vi "Find_ball.vi"(0 "Image Input":T1, 3 "error in (no error)":errorcluster) -> (4 "Image Out":T1(plugin-control), 5 "Plate coordinates":sgl[](array[numeric]), 6 "Ball Coordinates":cluster{"x":sgl, "y":sgl}, 7 "error out":errorcluster)   [LabVIEW 2021]
uses:
  <vilib>/vision/Image Controls.llb/IMAQ Image.ctl
  <vilib>/vision/NI_Vision_Development_Module.lvlib
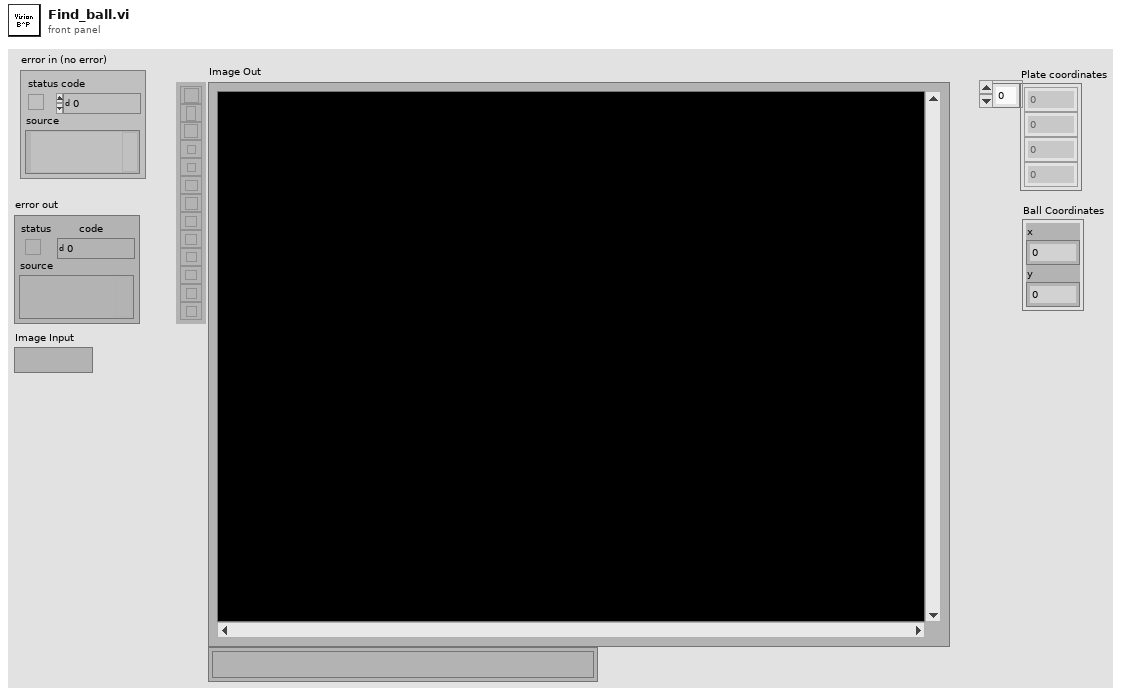
[diagram p1: front panel]
types:
  T1 = typedef "IMAQ Image.ctl" = refnum<image>
  T2 = cluster{"Feature":u32, "Points IDs":cluster{"GUID":string, "Index":i32}[]}[]
  T3 = typedef "Image Type" = u32
  T4 = cluster{"Global Rectangle":i32[], "Contours":cluster{"ID":enum32{"External", "Internal"}, "Type":u32, "Coordinates":i32[]}[]}
  T5 = cluster{"Show Search Area":bool, "Show Search Lines":bool, "Show Edges Found":bool, "Show Result":bool}
  T6 = cluster{"Number of Lines":i32, "Type":enum32{"First Edge Rake", "Best Edge Rake", "Hough Edge Rake", "First Edge Projection", "Best Edge Projection"}, "Min. Score":dbl, "Max. Score":dbl, "Orientation":dbl, "Angle Range":dbl, "Angle Tolerance":dbl, "Step Size":u32, "Min. SNR (db)":dbl, "Min. Points (%)":dbl, "Hough Iterations":i32}
  T7 = cluster{"Edge Polarity":u32, "Kernel Size":u32, "Width":u32, "Minimum Edge Strength":sgl, "Interpolation Type":enum32{"Zero Order", "Bilinear", "Quadratic", "Cubic", "Bilinear Fixed"}, "Data Processing Method":enum32{"Average", "Median"}}
  T8 = cluster{"Origin Pixel":cluster{"X":sgl, "Y":sgl}, "X Axis Pixel":cluster{"X":sgl, "Y":sgl}, "Axis Reference":u32}
  T9 = cluster{"Point1 (Pixels)":cluster{"X":sgl, "Y":sgl}, "Point2 (Pixels)":cluster{"X":sgl, "Y":sgl}, "Point1 (Real-World)":cluster{"X":sgl, "Y":sgl}, "Point2 (Real-World)":cluster{"X":sgl, "Y":sgl}, "Angle (Pixel)":dbl, "Angle (Real-World)":dbl, "Score":dbl, "Straightness":dbl, "Average SNR (db)":dbl, "Calibration Valid":bool}[]
  T10 = typedef "Search Line.ctl" = cluster{"Start Point":cluster{"X":sgl, "Y":sgl}, "End Point":cluster{"X":sgl, "Y":sgl}, "Edge Info":T11[], "Edge Map":dbl[], "Calibration Valid":bool}
  T11 = typedef "Edge New.ctl" = cluster{"Location (Pixel)":cluster{"X":sgl, "Y":sgl}, "Location (Real-World)":cluster{"X":sgl, "Y":sgl}, "Distance (Pixel)":dbl, "Distance (Real-World)":dbl, "Strength":dbl, "Noise":dbl, "Rising?":bool}
  T12 = cluster{"Straight Edges":cluster{"Point1 (Pixels)":cluster{"X":sgl, "Y":sgl}, "Point2 (Pixels)":cluster{"X":sgl, "Y":sgl}, "Point1 (Real-World)":cluster{"X":sgl, "Y":sgl}, "Point2 (Real-World)":cluster{"X":sgl, "Y":sgl}, "Angle (Pixel)":dbl, "Angle (Real-World)":dbl, "Score":dbl, "Straightness":dbl, "Average SNR (db)":dbl, "Calibration Valid":bool}[], "Search Lines Information":T10[], "Used Edges":cluster{"Edge Information":T11[]}[]}
  T13 = cluster{"Position":cluster{"x":sgl, "y":sgl}, "Angle":sgl, "Scale":sgl, "Score":sgl, "Bounding Box":cluster{"x":sgl, "y":sgl}[]}[]
  T14 = cluster{"Position":cluster{"x":sgl, "y":sgl}, "Angle":sgl, "Scale":sgl, "Score":sgl, "Bounding Box":cluster{"x":sgl, "y":sgl}[]}
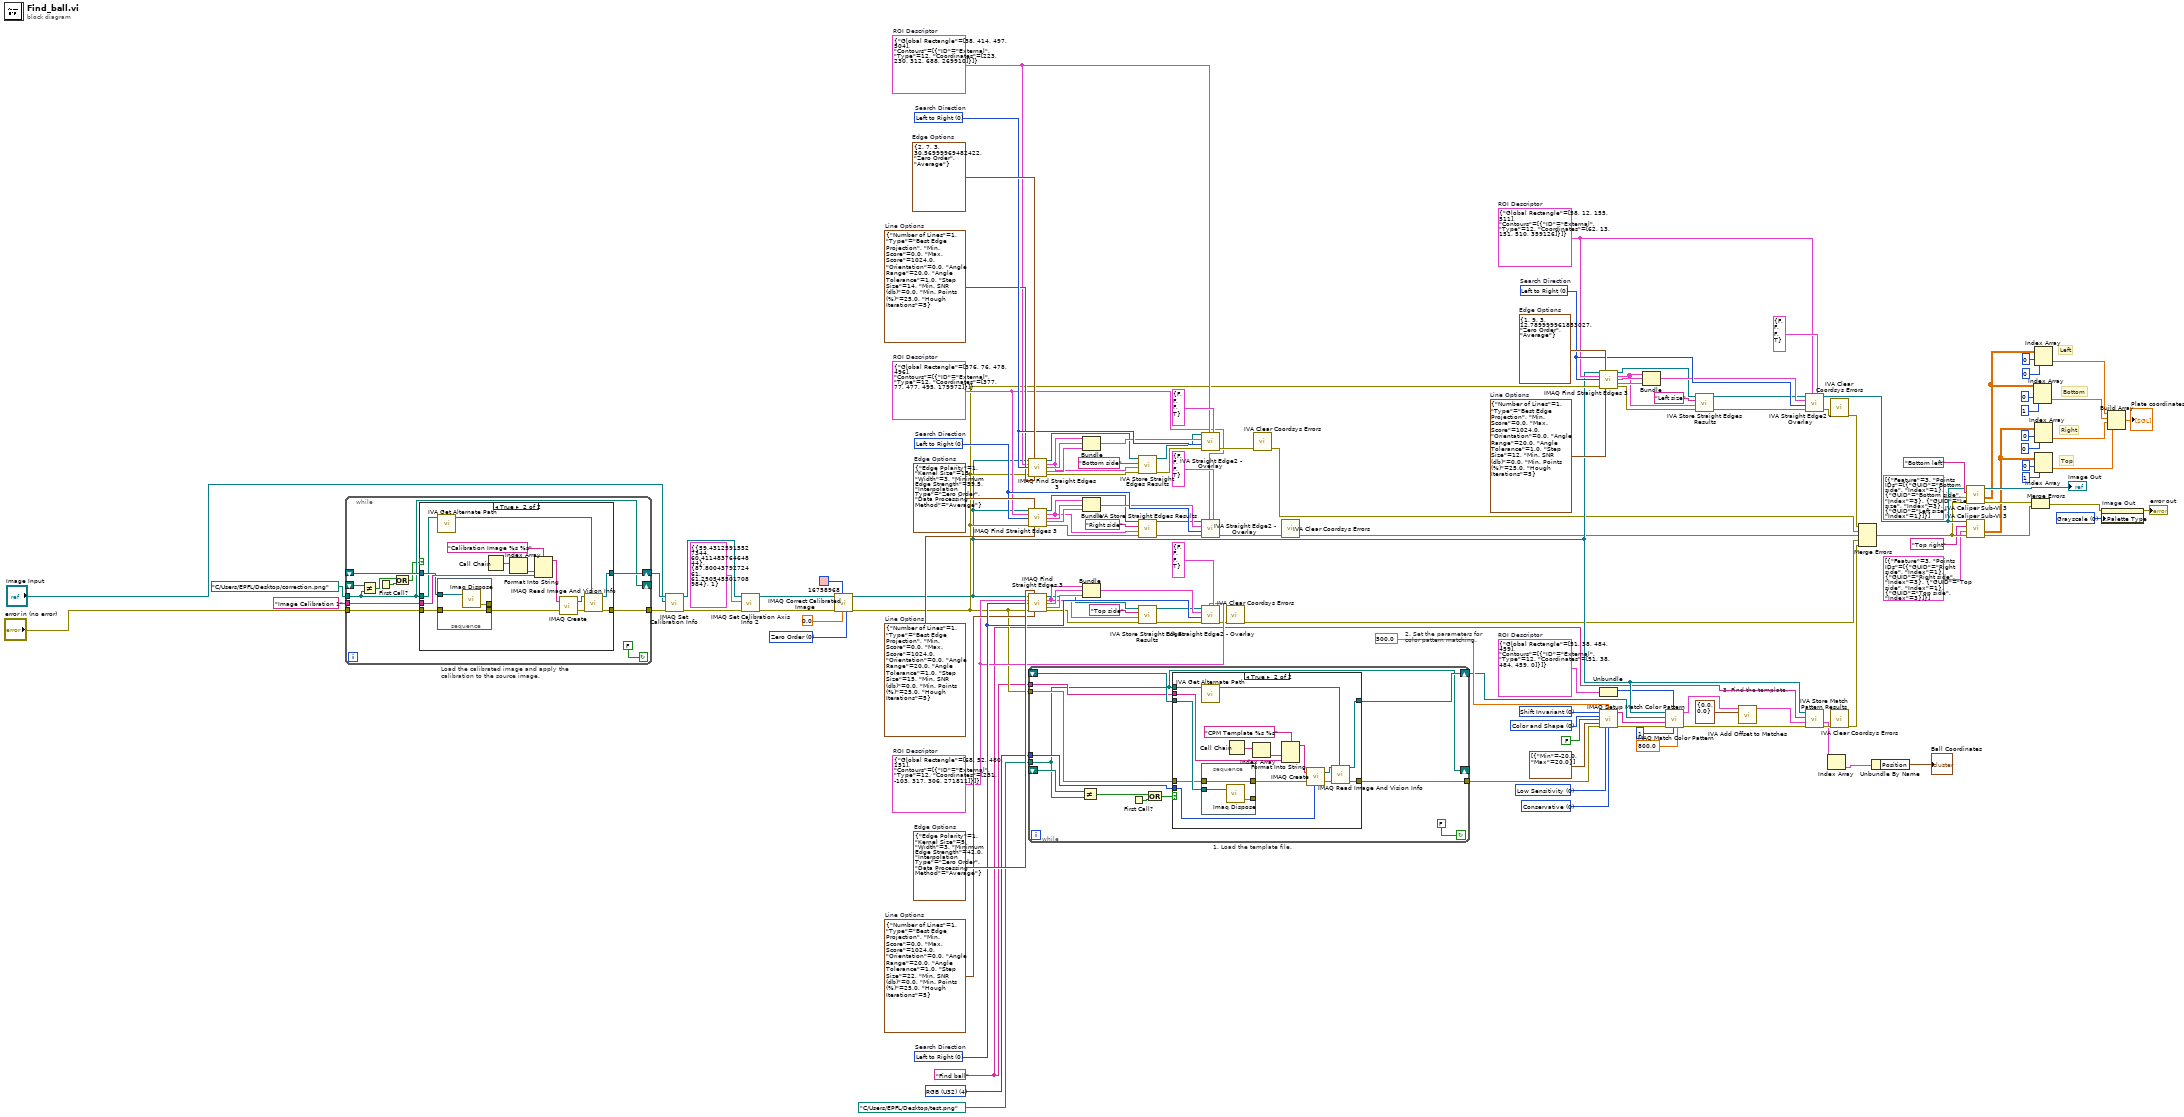
[diagram p0: block diagram]
diagram:
  w21 = u32 0 items=["Grayscale", "Binary", "Gradient", "Rainbow", "Temperature", "User Defined", "Binary 16 Bit", "Gradient 16 Bit", "Rainbow 16 Bit", "Temperature 16 Bit", "User Defined 16 Bit"] ("Palette Type")
  w45 = "Find ball" ("Step Name")
  w53 = T3 4 items=["Grayscale (U8)", "Grayscale (I16)", "Grayscale (SGL)", "Complex (CSG)", "RGB (U32)", "HSL (U32)", "RGB (U64)"] ("Image Type")
  w56 = u32 0 items=["Conservative", "Balance", "Aggressive", "Very Aggressive"] ("Search Strategy")
  w57 = u32 0 items=["Low Sensitivity", "Medium Sensitivity", "High Sensitivity"] ("Color Sensitivity")
  w59 = u32 0 items=["Color and Shape", "Color", "Shape"] ("Match Feature Mode")
  w60 = u32 0 items=["Shift Invariant", "Rotation Invariant"] ("Match Mode")
  w50 = T4 {"Global Rectangle"=[51, 38, 484, 459], "Contours"=[{"ID"=enum."External", "Type"=12, "Coordinates"=[51, 38, 484, 459, 0]}]}  # ROI Descriptor
  w75 = T6 {"Number of Lines"=1, "Type"=enum."Best Edge Projection", "Min. Score"=0.0, "Max. Score"=1024.0, "Orientation"=0.0, "Angle Range"=20.0, "Angle Tolerance"=1.0, "Step Size"=22, "Min. SNR (db)"=0.0, "Min. Points (%)"=25.0, "Hough Iterations"=5}  # Line Options
  w76 = u32 0 items=["Left to Right", "Right to Left", "Top to Bottom", "Bottom to Top"]  # Search Direction
  w77 = T7 {"Edge Polarity"=1, "Kernel Size"=5, "Width"=3, "Minimum Edge Strength"=42.0, "Interpolation Type"=enum."Zero Order", "Data Processing Method"=enum."Average"}  # Edge Options
  w70 = T4 {"Global Rectangle"=[68, 52, 480, 151], "Contours"=[{"ID"=enum."External", "Type"=12, "Coordinates"=[231, -103, 317, 306, 271811]}]}  # ROI Descriptor
  w90 = T6 {"Number of Lines"=1, "Type"=enum."Best Edge Projection", "Min. Score"=0.0, "Max. Score"=1024.0, "Orientation"=0.0, "Angle Range"=20.0, "Angle Tolerance"=1.0, "Step Size"=15, "Min. SNR (db)"=0.0, "Min. Points (%)"=25.0, "Hough Iterations"=5}  # Line Options
  w91 = u32 0 items=["Left to Right", "Right to Left", "Top to Bottom", "Bottom to Top"]  # Search Direction
  w92 = T7 {"Edge Polarity"=1, "Kernel Size"=15, "Width"=3, "Minimum Edge Strength"=59.5, "Interpolation Type"=enum."Zero Order", "Data Processing Method"=enum."Average"}  # Edge Options
  w85 = T4 {"Global Rectangle"=[376, 76, 478, 496], "Contours"=[{"ID"=enum."External", "Type"=12, "Coordinates"=[377, 77, 477, 495, 179972]}]}  # ROI Descriptor
  w105 = T6 {"Number of Lines"=1, "Type"=enum."Best Edge Projection", "Min. Score"=0.0, "Max. Score"=1024.0, "Orientation"=0.0, "Angle Range"=20.0, "Angle Tolerance"=1.0, "Step Size"=14, "Min. SNR (db)"=0.0, "Min. Points (%)"=25.0, "Hough Iterations"=5}  # Line Options
  w106 = u32 0 items=["Left to Right", "Right to Left", "Top to Bottom", "Bottom to Top"]  # Search Direction
  w107 = T7 {"Edge Polarity"=2, "Kernel Size"=7, "Width"=3, "Minimum Edge Strength"=30.57, "Interpolation Type"=enum."Zero Order", "Data Processing Method"=enum."Average"}  # Edge Options
  w100 = T4 {"Global Rectangle"=[38, 414, 497, 504], "Contours"=[{"ID"=enum."External", "Type"=12, "Coordinates"=[223, 230, 312, 688, 269910]}]}  # ROI Descriptor
  w120 = T6 {"Number of Lines"=1, "Type"=enum."Best Edge Projection", "Min. Score"=0.0, "Max. Score"=1024.0, "Orientation"=0.0, "Angle Range"=20.0, "Angle Tolerance"=1.0, "Step Size"=12, "Min. SNR (db)"=0.0, "Min. Points (%)"=25.0, "Hough Iterations"=5}  # Line Options
  w121 = u32 0 items=["Left to Right", "Right to Left", "Top to Bottom", "Bottom to Top"]  # Search Direction
  w122 = T7 {"Edge Polarity"=1, "Kernel Size"=9, "Width"=3, "Minimum Edge Strength"=12.79, "Interpolation Type"=enum."Zero Order", "Data Processing Method"=enum."Average"}  # Edge Options
  w115 = T4 {"Global Rectangle"=[58, 12, 155, 511], "Contours"=[{"ID"=enum."External", "Type"=12, "Coordinates"=[62, 13, 151, 510, 359126]}]}  # ROI Descriptor
  w127 = u32 0 items=["Zero Order", "Bi-Linear", "Quadratic", "Cubic Spline"] ("Interpolation Type")
  # "Top"
  # "Right"
  # "Bottom"
  # "Left"
  # "2. Set the parameters for\ncolor pattern matching."
  # "3. Find the template."
  n1 = while "Load the calibrated image and apply the calibration to the source image." {
    shift-right: [w145] -> w133
    shift-left: _ -> [w144]
    tunnel: [w142] -> w132
    tunnel: "error in (no error)" -> [w141]
    tunnel: path "C:/Users/EPFL/Desktop/correction.png" ("File Path") -> [w138]
    tunnel: "Image Calibration 1" ("Step Name") -> [w140]
    shift-right: [w138] -> _
    shift-left: _ -> [w139]
    stop <- FALSE continue-if-true
    n2 = Not Equal?(x=w139, y=w138) -> (x != y?=w136:bool)
    n3 = First Call?() -> (First Call?: T/F=w137:bool)
    n4 = Or(x=w136, y=w137) -> (x .or. y?=w135:bool)
    n5 = case shown="True" w135 {
      tunnel: [w147 w159] -> w145
      tunnel: w144 -> [w147 w151]
      tunnel: [w146 w156] -> w142
      tunnel: w141 -> [w146 w152]
      tunnel: w138 -> [_ w149]
      tunnel: w140 -> [_ w153]
      frame False {
      }
      frame True {
        n6 = call <vilib>:"IVA Get Alternate Path.vi"("Path In"=w149) -> ("Path Out"=w148:path)  [unwired: 10 out]
        n7 = stacked-sequence {
          tunnel: w152 -> [w163]
          tunnel: w151 -> [w164]
          tunnel: [w163] -> w150
          tunnel: [w162] -> _
          frame #0 {
            n8 = call "Imaq Dispose"("Image"=w164) -> ("error out"=w162:errorcluster)  [unwired: 2 in, 3 out]
          }
        }
        n9 = Call Chain() -> (call chain=w155:string[])
        n10 = Index Array(array=w155) -> (element=w154:string)  [unwired: 1 in]
        n11 = Format Into String(format string="Calibration Image %s %s" ("Image Name"), w154, w153) -> (resulting string=w161:string)  [unwired: 2 in, 1 out]
        n12 = call "IMAQ Create"("Image Name"=w161, "error in (no error)"=w150) -> ("New Image"=w158:T1, "error out"=w157:errorcluster)  [unwired: 2 in, 1 out]
        n13 = call "IMAQ Read Image And Vision Info"("File Path"=w148, "error in (no error)"=w157, "Image"=w158) -> ("error out"=w156:errorcluster, "Image Out"=w159:T1)  [unwired: 1 in, 6 out]
      }
    }
  }
  n14 = call "IMAQ Set Calibration Info"("error in (no error)"=w132, "Image Dst"="Image Input", "Image Src"=w133) -> ("error out"=w129:errorcluster, "Calibrated Image"=w130:T1)  [unwired: 1 in, 6 out]
  n15 = call-poly "IMAQ Set Calibration Axis Info 2"("error in (no error)"=w129, "Calibration Axis Info"=T8 {"Origin Pixel"={"X"=59.43126, "Y"=60.411484}, "X Axis Pixel"={"X"=87.80044, "Y"=61.250546}, "Axis Reference"=1}, "Calibration Template Image In"=w130) -> ("error out"=w125:errorcluster, "Calibration Template Image Out"=w126:T1)  [unwired: 7 out]
  n16 = call "IMAQ Correct Calibrated Image"("Interpolation Type"=w127, "Replace Value"=sgl 0.0, "Color Replace Value"=u32 16758968, "error in (no error)"=w125, "Image Src"=w126) -> ("error out"=w49:errorcluster, "Corrected Image"=w46:T1)  [unwired: 2 in, 3 out]
  n17 = call "IMAQ Find Straight Edges 3"("Image"=w46, "Edge Options"=w107, "ROI Descriptor"=w100, "Search Direction"=w106, "error in (no error)"=w49, "Line Options"=w105) -> ("Image (duplicate)"=w97:T1, "Straight Edges"=w98:T9, "Search Lines Information"=w102:T10[], "Used Edges"=w103:cluster{"Edge Information":T11[]}[], "error out"=w95:errorcluster)  [unwired: 1 in, 4 out]
  n18 = call "IMAQ Find Straight Edges 3"("Image"=w46, "Edge Options"=w92, "ROI Descriptor"=w85, "Search Direction"=w91, "error in (no error)"=w49, "Line Options"=w90) -> ("Image (duplicate)"=w82:T1, "Straight Edges"=w83:T9, "Search Lines Information"=w87:T10[], "Used Edges"=w88:cluster{"Edge Information":T11[]}[], "error out"=w80:errorcluster)  [unwired: 1 in, 4 out]
  n19 = call "IMAQ Find Straight Edges 3"("Image"=w46, "Edge Options"=w77, "ROI Descriptor"=w70, "Search Direction"=w76, "error in (no error)"=w49, "Line Options"=w75) -> ("Image (duplicate)"=w67:T1, "Straight Edges"=w68:T9, "Search Lines Information"=w72:T10[], "Used Edges"=w73:cluster{"Edge Information":T11[]}[], "error out"=w65:errorcluster)  [unwired: 1 in, 4 out]
  n20 = while "1. Load the template file." {
    shift-right: [w176] -> w40
    shift-left: _ -> [w175]
    tunnel: [w173] -> w39
    tunnel: w49 -> [w172]
    tunnel: path "C:/Users/EPFL/Desktop/test.png" ("File Path") -> [w168]
    tunnel: w53 -> [w171]
    tunnel: w45 -> [w170]
    shift-right: [w168] -> _
    shift-left: _ -> [w169]
    stop <- FALSE continue-if-true
    n21 = Not Equal?(x=w169, y=w168) -> (x != y?=w166:bool)
    n22 = First Call?() -> (First Call?: T/F=w167:bool)
    n23 = Or(x=w166, y=w167) -> (x .or. y?=w165:bool)
    n24 = case shown="True" w165 {
      tunnel: [w178 w191] -> w176
      tunnel: w175 -> [w178 w183]
      tunnel: [w177 w188] -> w173
      tunnel: w172 -> [w177 w182]
      tunnel: w168 -> [_ w180]
      tunnel: w171 -> [_ w187]
      tunnel: w170 -> [_ w184]
      frame False {
      }
      frame True {
        n25 = call <vilib>:"IVA Get Alternate Path.vi"("Path In"=w180) -> ("Path Out"=w179:path)  [unwired: 10 out]
        n26 = stacked-sequence {
          tunnel: w183 -> [w196]
          tunnel: w182 -> [w195]
          tunnel: [w195] -> w181
          tunnel: [w194] -> _
          frame #0 {
            n27 = call "Imaq Dispose"("Image"=w196) -> ("error out"=w194:errorcluster)  [unwired: 2 in, 3 out]
          }
        }
        n28 = Call Chain() -> (call chain=w186:string[])
        n29 = Index Array(array=w186) -> (element=w185:string)  [unwired: 1 in]
        n30 = Format Into String(format string="CPM Template %s %s" ("Image Name"), w185, w184) -> (resulting string=w193:string)  [unwired: 2 in, 1 out]
        n31 = call "IMAQ Create"("Image Name"=w193, "Image Type"=w187, "error in (no error)"=w181) -> ("New Image"=w190:T1, "error out"=w189:errorcluster)  [unwired: 1 in, 1 out]
        n32 = call "IMAQ Read Image And Vision Info"("File Path"=w179, "error in (no error)"=w189, "Image"=w190) -> ("error out"=w188:errorcluster, "Image Out"=w191:T1)  [unwired: 1 in, 6 out]
      }
    }
  }
  n33 = Bundle("Straight Edges"=w98, "Search Lines Information"=w102, "Used Edges"=w103) -> (w99:T12)  [unwired: 1 out]
  n34 = Bundle("Straight Edges"=w83, "Search Lines Information"=w87, "Used Edges"=w88) -> (w84:T12)  [unwired: 1 out]
  n35 = Bundle("Straight Edges"=w68, "Search Lines Information"=w72, "Used Edges"=w73) -> (w69:T12)  [unwired: 1 out]
  n36 = call <vilib>:"IVA Store Straight Edges Results.vi"("error in (no error)"=w95, "Straight Edges"=w98, "Step Name"="Bottom side", "Image in"=w97) -> ("error out"=w94:errorcluster, "Image dup"=w96:T1)  [unwired: 6 out]
  n37 = call <vilib>:"IVA Store Straight Edges Results.vi"("error in (no error)"=w80, "Straight Edges"=w83, "Step Name"="Right side", "Image in"=w82) -> ("error out"=w79:errorcluster, "Image dup"=w81:T1)  [unwired: 6 out]
  n38 = call <vilib>:"IVA Store Straight Edges Results.vi"("error in (no error)"=w65, "Straight Edges"=w68, "Step Name"="Top side", "Image in"=w67) -> ("error out"=w64:errorcluster, "Image dup"=w66:T1)  [unwired: 6 out]
  n39 = call <vilib>:"IVA Straight Edge2 - Overlay.vi"("Setup"=T5 {"Show Search Area"=FALSE, "Show Search Lines"=FALSE, "Show Edges Found"=FALSE, "Show Result"=TRUE}, "Search Area"=w100, "error in (no error)"=w94, "Scan Direction"=w106, "Edge Results"=w99, "Image In"=w96) -> ("error out"=w93:errorcluster)  [unwired: 1 in, 4 out]
  n40 = call <vilib>:"IVA Straight Edge2 - Overlay.vi"("Setup"=T5 {"Show Search Area"=FALSE, "Show Search Lines"=FALSE, "Show Edges Found"=FALSE, "Show Result"=TRUE}, "Search Area"=w85, "error in (no error)"=w79, "Scan Direction"=w91, "Edge Results"=w84, "Image In"=w81) -> ("error out"=w78:errorcluster)  [unwired: 1 in, 4 out]
  n41 = call <vilib>:"IVA Straight Edge2 - Overlay.vi"("Setup"=T5 {"Show Search Area"=FALSE, "Show Search Lines"=FALSE, "Show Edges Found"=FALSE, "Show Result"=TRUE}, "Search Area"=w70, "error in (no error)"=w64, "Scan Direction"=w76, "Edge Results"=w69, "Image In"=w66) -> ("error out"=w63:errorcluster)  [unwired: 1 in, 4 out]
  n42 = call <vilib>:"IVA Clear Coordsys Errors.vi"("error in (no error)"=w63) -> ("error out"=w34:errorcluster)  [unwired: 10 in]
  n43 = call <vilib>:"IVA Clear Coordsys Errors.vi"("error in (no error)"=w93) -> ("error out"=w36:errorcluster)  [unwired: 10 in]
  n44 = call <vilib>:"IVA Clear Coordsys Errors.vi"("error in (no error)"=w78) -> ("error out"=w35:errorcluster)  [unwired: 10 in]
  n45 = call "IMAQ Find Straight Edges 3"("Image"=w46, "Edge Options"=w122, "ROI Descriptor"=w115, "Search Direction"=w121, "error in (no error)"=w49, "Line Options"=w120) -> ("Image (duplicate)"=w112:T1, "Straight Edges"=w113:T9, "Search Lines Information"=w117:T10[], "Used Edges"=w118:cluster{"Edge Information":T11[]}[], "error out"=w110:errorcluster)  [unwired: 1 in, 4 out]
  n46 = Unbundle(w50) -> ("Global Rectangle"=w41:i32[])  [unwired: 1 out]
  n47 = call "IMAQ Setup Match Color Pattern"("Match Mode"=w60, "Color Score Weight"=sgl 500.0, "Match Feature Mode"=w59, "Subpixel Accuracy"=FALSE, "Rotation Angle Ranges (degrees)"=cluster{"Min":sgl, "Max":sgl}[] [{"Min"=-20.0, "Max"=20.0}], "error in (no error)"=w39, "Color Sensitivity"=w57, "Search Strategy"=w56) -> ("Match Color Pattern Setup Data"=w44:string, "error out"=w43:errorcluster)  [unwired: 1 in, 5 out]
  n48 = Bundle("Straight Edges"=w113, "Search Lines Information"=w117, "Used Edges"=w118) -> (w114:T12)  [unwired: 1 out]
  n49 = call "IMAQ Match Color Pattern"("Minimum Match Score"=sgl 800.0, "Number of Matches Requested"=1, "Optional Rectangle"=w41, "error in (no error)"=w43, "Match Color Pattern Setup Data"=w44, "Template Image"=w40, "Image"=w46) -> ("error out"=w47:errorcluster, "Matches"=w42:T13)  [unwired: 3 out]
  n50 = call <vilib>:"IVA Store Straight Edges Results.vi"("error in (no error)"=w110, "Straight Edges"=w113, "Step Name"="Left size", "Image in"=w112) -> ("error out"=w109:errorcluster, "Image dup"=w111:T1)  [unwired: 6 out]
  n51 = call <vilib>:"IVA Add Offset to Matches.vi"("Match Offset"=cluster{"X":sgl, "Y":sgl} {"X"=0.0, "Y"=0.0}, "Matches in"=w42) -> ("Matches out"=w48:T13)  [unwired: 9 out]
  n52 = call <vilib>:"IVA Straight Edge2 - Overlay.vi"("Setup"=T5 {"Show Search Area"=FALSE, "Show Search Lines"=FALSE, "Show Edges Found"=FALSE, "Show Result"=TRUE}, "Search Area"=w115, "error in (no error)"=w109, "Scan Direction"=w121, "Edge Results"=w114, "Image In"=w111) -> ("error out"=w108:errorcluster, "Image Out"=w30:T1)  [unwired: 1 in, 3 out]
  n53 = call <vilib>:"IVA Store Match Pattern Results.vi"("error in (no error)"=w47, "Matches"=w48, "Step Name"=w45, "Image in"=w46) -> ("error out"=w38:errorcluster, "Calibrated Matches"=w5:T13)  [unwired: 6 out]
  n54 = Index Array(array=w5) -> (element=w3:T14)  [unwired: 1 in]
  n55 = call <vilib>:"IVA Clear Coordsys Errors.vi"("error in (no error)"=w108) -> ("error out"=w37:errorcluster)  [unwired: 10 in]
  n56 = call <vilib>:"IVA Clear Coordsys Errors.vi"("error in (no error)"=w38) -> ("error out"=w33:errorcluster)  [unwired: 10 in]
  n57 = Merge Errors(w37, w36, w35, w34, w33) -> (w29:errorcluster)
  n58 = Unbundle By Name(w3) -> ("Position"=→"Ball Coordinates":cluster{"x":sgl, "y":sgl})
  n59 = call <vilib>:"IVA Caliper Sub-VI 3.vi"("error in"=w29, "Parameters"=T2 [{"Feature"=3, "Points IDs"=[{"GUID"="Bottom side", "Index"=1}, {"GUID"="Bottom side", "Index"=3}, {"GUID"="Left size", "Index"=3}, {"GUID"="Left size", "Index"=1}]}], "Step Name"="Bottom left", "Image In"=w30) -> ("error out"=w26:errorcluster, "Results (Calibrated)"=w20:sgl[][], "Image Out"=→"Image Out":T1)  [unwired: 1 in, 4 out]
  n60 = call <vilib>:"IVA Caliper Sub-VI 3.vi"("error in"=w29, "Parameters"=T2 [{"Feature"=3, "Points IDs"=[{"GUID"="Right side", "Index"=1}, {"GUID"="Right side", "Index"=3}, {"GUID"="Top side", "Index"=1}, {"GUID"="Top side", "Index"=3}]}], "Step Name"="Top right", "Image In"=w30) -> ("error out"=w25:errorcluster, "Results (Calibrated)"=w13:sgl[][])  [unwired: 1 in, 5 out]
  n61 = Merge Errors(w26, w25) -> (w24:errorcluster)
  n62 = Index Array(array=w20, index (row)=0, index (col)=1 ("disabled index (col)")) -> (element=w14:sgl)
  n63 = Index Array(array=w13, index (row)=0, index (col)=0 ("disabled index (col)")) -> (element=w8:sgl)
  n64 = Index Array(array=w20, index (row)=0, index (col)=0 ("disabled index (col)")) -> (element=w15:sgl)
  n65 = Index Array(array=w13, index (row)=0, index (col)=1 ("disabled index (col)")) -> (element=w7:sgl)
  n66 = property on="Image Out" class="ImageControl"(error in=w24, "Palette:Palette Type"=w21) -> (error out=→"error out":errorcluster)  [unwired: 1 in, 1 out]
  n67 = Build Array(w15, w14, w8, w7) -> (→"Plate coordinates":sgl[])
